vi "1B_AnalyzePulseTrain.vi"(0 "Waveform In":waveform(dbl)={"t0"=timestamp(3433165898.5470004 s since 1904-01-01), "dt"=1e-05, "Y"=array[4250 elements]}, 5 "Repetitions in the Input Waveform":i32, 7 "Pulse Characteristics":T1={"Pulses per Cycle"=2, "Load Resistance (Ohms)"=750.0, "Krec Value"=2, "Recovery Mode (T=Active)"=TRUE, "Target Stim Currents (Amps)"=[]}) -> (2 "Avg. CBC Width":dbl format="%0.2f", 3 "Avg. CBC Amplitude":dbl format="%0.2f", 4 "Stim PW":dbl[](array[numeric]), 6 "Stim Amplitude":dbl[](array[numeric]), 8 "Interphase Delay":dbl[](array[numeric]), 10 "Recovery PW":dbl[](array[numeric]), 12 "Waveform Parameters":T2, 13 "Frequency":dbl, 14 "Recovery Holdoff":dbl[](array[numeric]), 15 "Recovery Amplitude":dbl[](array[numeric]))   [LabVIEW 2010]
uses:
  <vilib>/measure/mamon.llb/Trigger Detection for 1 Channel.vi
  <vilib>/measure/NI_MAPro.lvlib
  <vilib>/Analysis/NI_AALBase.lvlib
panel:
  in  "View":enum32{"View All", "Graph Only"}(tab)
  out "Waveform in ( graph )":waveform(dbl)(graph)
  out "Normalized Waveform":waveform(dbl)(graph)
  out "Offset":dbl
  out "Current in amps":waveform(dbl)(graph)
  # "Remove idle voltage offset\n( if applicable )"
  # "The input waveform should be a capture of the STIM chip output\n(before the cap) when the output is held at 1/2 HVDD by the\nLoad Resistance.  This ensures that passive recovery and CBC\npulses are captured, because they look like pulses pulled to GND."
  # "The elements in these arrays correspond to the pulses per cycle.\nThey are the averages over all the repetitions in the waveform."
  # "Enter Target Current\nfor each in array below"
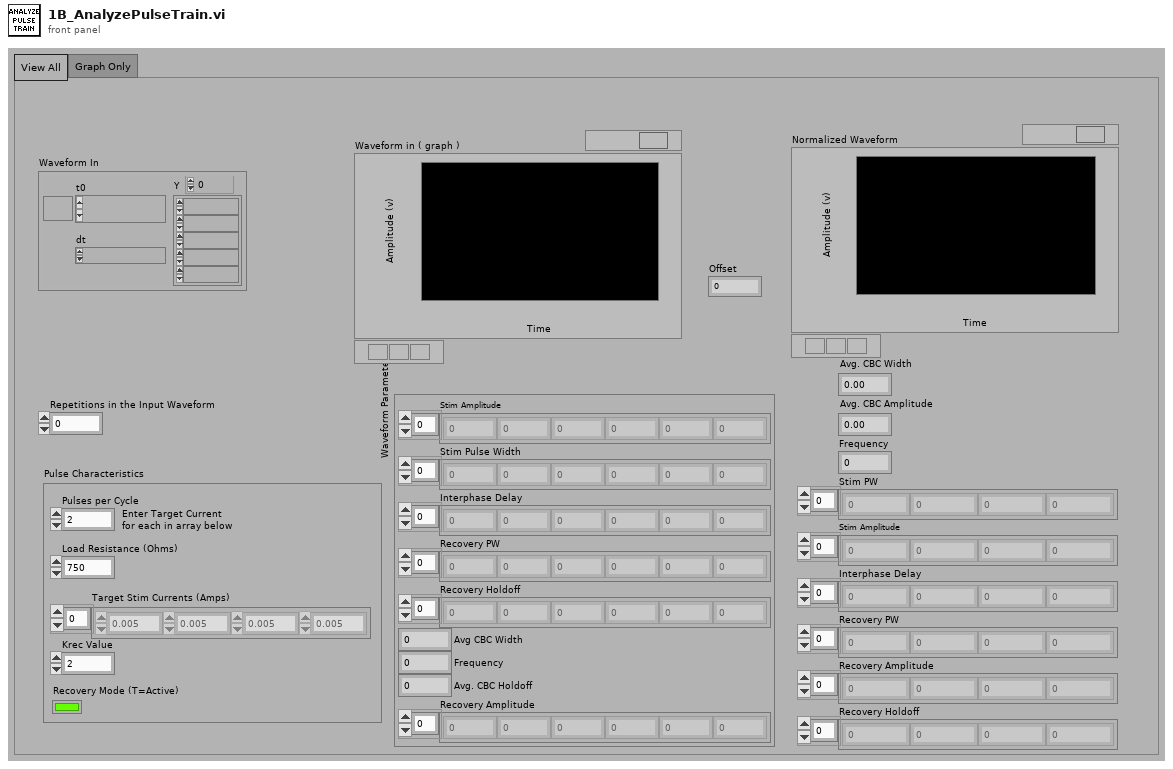
[diagram p1: front panel]
types:
  T1 = cluster{"Pulses per Cycle":i32, "Load Resistance (Ohms)":dbl, "Krec Value":i32, "Recovery Mode (T=Active)":bool, "Target Stim Currents (Amps)":dbl[]}
  T2 = cluster{"Stim Amplitude":dbl[], "Stim Pulse Width":dbl[], "Interphase Delay":dbl[], "Recovery PW":dbl[], "Recovery Holdoff":dbl[], "Avg CBC Width":dbl, "Frequency":dbl, "Avg. CBC Holdoff":dbl, "Recovery Amplitude":dbl[]}
  T3 = cluster{"trigger slope":u16, "Trigger Level":dbl}[]
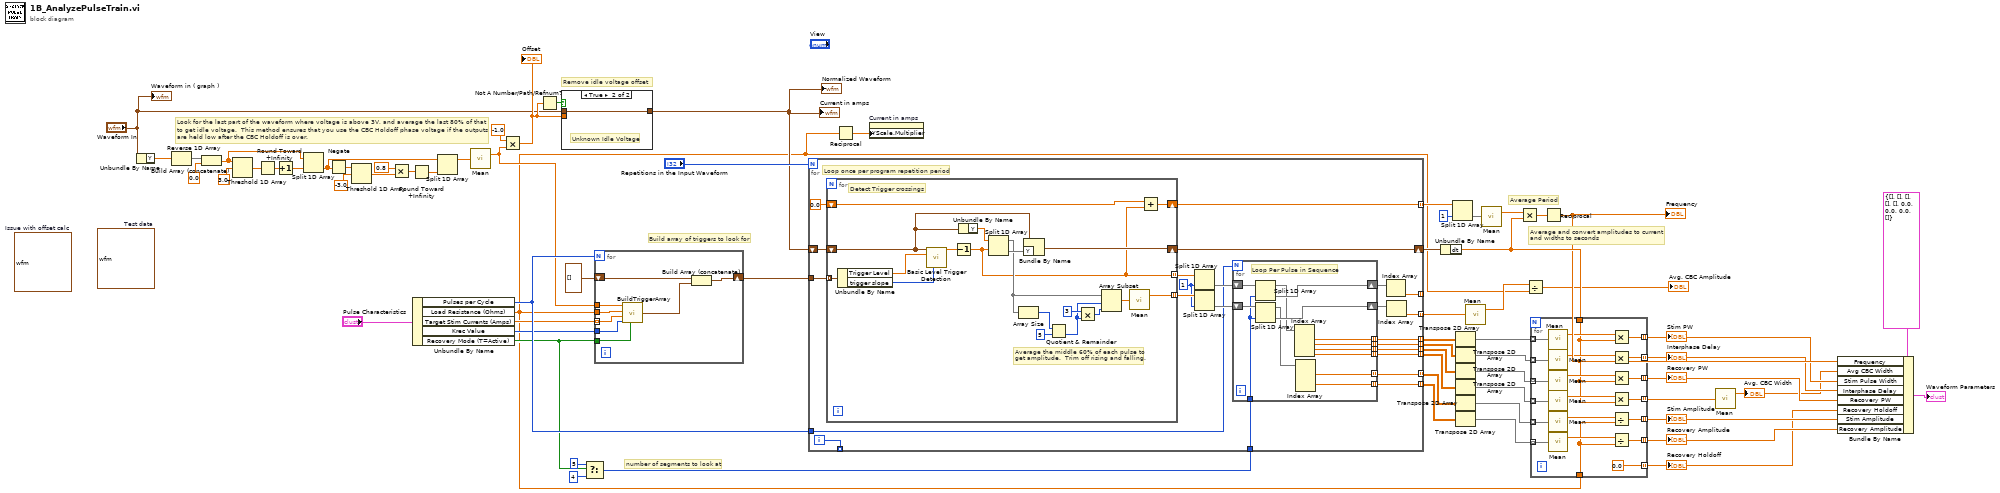
[diagram p0: block diagram]
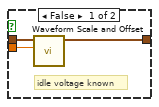
[diagram p2: hidden frame]
diagram:
  (unwired) waveform(dbl) {"t0"=timestamp(3458836317.3280005 s since 1904-01-01), "dt"=1.428e-05, "Y"=array[4000 elements]}  # Issue with offset calc
  (unwired) waveform(dbl) {"t0"=timestamp(3418839276.250478 s since 1904-01-01), "dt"=1e-06, "Y"=[5.0, 5.0, 9.0, 9.0, 9.0, 9.0, 9.0, 9.0, 9.0, 9.0, 5.0, 5.0, 5.0, 3.0, 3.0, 3.0, 3.0, 3.0, 3.0, 3.0, 3.0, 3.0, 3.0, 3.0, 3.0, 3.0, 3.0, 3.0, 3.0, 5.0, 5.0, 5.0, 5.0, 8.0, 8.0, 8.0, 8.0, 8.0, 8.0, 8.0, 8.0, 5.0, 5.0, 5.0, 3.0, 3.0, 3.0, 3.0, 3.0, 3.0, 3.0, 3.0, 3.0, 3.0, 3.0, 3.0, 3.0, 3.0, 3.0, 3.0, 5.0, 5.0, 5.0, 5.0, 0.0, 0.0, 0.0, 0.0, 0.0, 5.0, 5.0, 5.0, 5.0, 5.0, 5.0, 5.0, 5.0, 5.0, 5.0, 5.0, 5.0, 5.0, 5.0, 5.0, 5.0, 5.0, 5.0, 5.0, 5.0, 5.0, 5.0, 5.0, 5.0, 5.0, 5.0, 5.0, 5.0, 5.0, 5.0, 5.0, 5.0, 5.0, 9.0, 9.0, 9.0, 9.0, 9.0, 9.0, 9.0, 9.0, 5.0, 5.0, 5.0, 3.0, 3.0, 3.0, 3.0, 3.0, 3.0, 3.0, 3.0, 3.0, 3.0, 3.0, 3.0, 3.0, 3.0, 3.0, 3.0, 5.0, 5.0, 5.0, 5.0, 8.0, 8.0, 8.0, 8.0, 8.0, 8.0, 8.0, 8.0, 5.0, 5.0, 5.0, 3.0, 3.0, 3.0, 3.0, 3.0, 3.0, 3.0, 3.0, 3.0, 3.0, 3.0, 3.0, 3.0, 3.0, 3.0, 3.0, 5.0, 5.0, 5.0, 5.0, 0.0, 0.0, 0.0, 0.0, 0.0, 5.0, 5.0, 5.0, 5.0, 5.0, 5.0, 5.0, 5.0, 5.0, 5.0, 5.0, 5.0, 5.0, 5.0, 5.0, 5.0, 5.0, 5.0, 5.0, 5.0, 5.0, 5.0, 5.0, 5.0, 5.0, 5.0, 5.0, 5.0, 5.0, 5.0, 5.0, 5.0, 5.0, 9.0, 9.0, 9.0, 9.0, 9.0, 9.0, 9.0, 9.0, 5.0, 5.0, 5.0, 3.0, 3.0, 3.0, 3.0, 3.0, 3.0, 3.0, 3.0, 3.0, 3.0, 3.0, 3.0, 3.0, 3.0, 3.0, 3.0, 5.0, 5.0, 5.0, 5.0, 8.0, 8.0, 8.0, 8.0, 8.0, 8.0, 8.0, 8.0, 5.0, 5.0, 5.0, 3.0, 3.0, 3.0, 3.0, 3.0, 3.0, 3.0, 3.0, 3.0, 3.0, 3.0, 3.0, 3.0, 3.0, 3.0, 3.0, 5.0, 5.0, 5.0, 5.0, 0.0, 0.0, 0.0, 0.0, 0.0, 5.0, 5.0, 5.0, 5.0, 5.0, 5.0, 5.0, 5.0, 5.0, 5.0, 5.0, 5.0, 5.0, 5.0, 5.0, 5.0, 5.0, 5.0, 5.0, 5.0, 5.0, 5.0, 5.0, 5.0, 5.0, 5.0, 5.0, 5.0, 5.0, 5.0, 5.0, 5.0, 5.0, 9.0, 9.0, 9.0, 9.0, 9.0, 9.0, 9.0, 9.0, 5.0, 5.0, 5.0, 3.0, 3.0, 3.0, 3.0, 3.0, 3.0, 3.0, 3.0, 3.0, 3.0, 3.0, 3.0, 3.0, 3.0, 3.0, 3.0, 5.0, 5.0, 5.0, 5.0, 8.0, 8.0, 8.0, 8.0, 8.0, 8.0, 8.0, 8.0, 5.0, 5.0, 5.0, 3.0, 3.0, 3.0, 3.0, 3.0, 3.0, 3.0, 3.0, 3.0, 3.0, 3.0, 3.0, 3.0, 3.0, 3.0, 3.0, 5.0, 5.0, 5.0, 5.0, 0.0, 0.0, 0.0, 0.0, 0.0, 5.0, 5.0, 5.0, 5.0, 5.0, 5.0, 5.0, 5.0, 5.0, 5.0, 5.0, 5.0, 5.0, 5.0, 5.0, 5.0, 5.0, 5.0, 5.0, 5.0, 5.0, 5.0, 5.0, 5.0, 5.0, 5.0, 5.0, 5.0, 5.0, 5.0, 5.0, 5.0, 5.0, 9.0, 9.0, 9.0, 9.0, 9.0, 9.0, 9.0, 9.0, 5.0, 5.0, 5.0, 3.0, 3.0, 3.0, 3.0, 3.0, 3.0, 3.0, 3.0, 3.0, 3.0, 3.0, 3.0, 3.0, 3.0, 3.0, 3.0, 5.0, 5.0, 5.0, 5.0, 8.0, 8.0, 8.0, 8.0, 8.0, 8.0, 8.0, 8.0, 5.0, 5.0, 5.0, 3.0, 3.0, 3.0, 3.0, 3.0, 3.0, 3.0, 3.0, 3.0, 3.0, 3.0, 3.0, 3.0, 3.0, 3.0, 3.0, 5.0, 5.0, 5.0, 5.0, 0.0, 0.0, 0.0, 0.0, 0.0, 5.0, 5.0, 5.0, 5.0, 5.0, 5.0, 5.0, 5.0, 5.0, 5.0, 5.0, 5.0, 5.0, 5.0, 5.0, 5.0, 5.0, 5.0, 5.0, 5.0, 5.0, 5.0, 5.0, 5.0, 5.0, 5.0, 5.0, 5.0, 5.0, 5.0, 5.0, 5.0, 5.0, 5.0]}  # Test data
  # "number of segments to look at"
  # "Look for the last part of the waveform where voltage is above 3V, and average the last 80% of that\nto get idle voltage.  This method ensures that you use the CBC Holdoff phase voltage if the outputs\nare held low after the CBC Holdoff is over."
  # "Average Period"
  # "Average and convert amplitudes to current\nand widths to seconds"
  # "Build array of triggers to look for"
  # "Remove idle voltage offset"
  n1 = Unbundle By Name("Waveform In") -> ("Y"=w2:dbl[])
  n2 = Reverse 1D Array(array=w2) -> (reversed array=w31:dbl[])
  n3 = Build Array (concatenate)(w31, 0.0 ("y")) -> (w5:dbl[])
  n4 = Threshold 1D Array(2:3.0 ("y"), 3:w5) -> (0:w28:dbl)  [unwired: 1 in]
  n5 = Round Toward +Infinity(x=w28) -> (ceil(x): smallest int >= x=w27:dbl)
  n6 = Increment(x=w27) -> (x+1=w20:dbl)
  n7 = Split 1D Array(array=w5, index=w20) -> (second subarray=w4:dbl[])  [unwired: 1 out]
  n8 = Negate(x=w4) -> (-x=w25:dbl[])
  n9 = Threshold 1D Array(2:-3.0 ("y"), 3:w25) -> (0:w24:dbl)  [unwired: 1 in]
  n10 = Multiply(x=0.8, y=w24) -> (x*y=w22:dbl)
  n11 = Round Toward +Infinity(x=w22) -> (ceil(x): smallest int >= x=w21:dbl)
  n12 = Unbundle By Name("Pulse Characteristics") -> ("Pulses per Cycle"=w52:i32, "Load Resistance (Ohms)"=w9:dbl, "Target Stim Currents (Amps)"=w51:dbl[], "Krec Value"=w50:i32, "Recovery Mode (T=Active)"=w14:bool)
  n13 = Split 1D Array(array=w4, index=w21) -> (first subarray=w3:dbl[])  [unwired: 1 out]
  n14 = call <vilib>:"Mean.vi"("X"=w3) -> ("mean"=w15:dbl)  [unwired: 1 out]
  n15 = Multiply(x=-1.0, y=w15) -> (x*y=w7:dbl)
  "Offset" <- w7
  n16 = Not A Number/Path/Refnum?(number/path/refnum=w7) -> (NaN/Path/Refnum?=w6:bool)
  n17 = case shown="True" w6 {
    tunnel: [w71 w72] -> w10
    tunnel: "Waveform In" -> [w70 w72]
    tunnel: w7 -> [w69 _]
    frame False {
      # "idle voltage known"
      n18 = call <vilib>:"Waveform Scale and Offset.vi"("offset"=w69, "waveform in"=w70) -> ("waveform out"=w71:waveform(dbl))  [unwired: 8 in, 1 out]
    }
    frame True {
      # "Unknown Idle Voltage"
    }
  }
  "Normalized Waveform" <- w10
  "Current in amps" <- w10
  n19 = Select(t=5, s=w14, f=4 ("index")) -> (s? t:f=w12:i32)
  n20 = for {
    N: w52 -> [_]
    shift-right: [w80] -> w19
    shift-left: T3 [] -> [w79]
    tunnel: w15 -> [w78]
    tunnel: w14 -> [w77]
    tunnel: w9 -> [w76]
    tunnel: w51 -> [w75] mode=indexing
    tunnel: w50 -> [w74]
    n21 = call "BuildTriggerArray.vi"("CBC Trigger Level"=w78, "Load Resistance (Ohms)"=w76, "Target Stim Current (Amps)"=w75, "Krec Value"=w74, "Recovery Mode (T=Active)"=w77) -> ("Pulse Triggers"=w73:T3)
    n22 = Build Array (concatenate)(w79, w73) -> (w80:T3)
  }
  n23 = for {
    N: "Repetitions in the Input Waveform" -> [_]
    tunnel: w19 -> [w103]
    shift-right: [w99] -> w48
    shift-left: w10 -> [w102]
    tunnel: w52 -> [w96]
    tunnel: [w93] -> _ mode=indexing
    tunnel: [w92] -> w65 mode=indexing
    tunnel: [w91] -> w64 mode=indexing
    tunnel: [w90] -> w63 mode=indexing
    tunnel: [w89] -> w62 mode=indexing
    tunnel: [w88] -> w61 mode=indexing
    tunnel: [w87] -> w60 mode=indexing
    tunnel: [w86] -> w59 mode=indexing
    tunnel: [w83] -> w46 mode=indexing
    tunnel: w12 -> [w82]
    tunnel: [w81] -> _ mode=indexing
    i -> [w81]
    w100 = 1 ("index")
    # "Loop once per program repetition period"
    n24 = for {
      tunnel: w103 -> [w135] mode=indexing
      shift-right: [w121] -> w99
      shift-left: w102 -> [w130]
      tunnel: [w122] -> w101 mode=indexing
      tunnel: [w117] -> w84 mode=indexing
      shift-right: [w120] -> w83
      shift-left: 0.0 -> [w119]
      # "Detect Trigger crossings"
      # "Average the middle 60% of each pulse to\nget amplitude.  Trim off rising and falling."
      n25 = Unbundle By Name(w135) -> ("Trigger Level"=w134:dbl, "trigger slope"=w133:u16)
      n26 = call-poly <vilib>:"Basic Level Trigger Detection.vi"("signal in"=w130, "level"=w134, "trigger slope"=w133) -> ("trigger location"=w118:dbl)  [unwired: 10 in, 2 out]
      n27 = Decrement(x=w118) -> (x-1=w117:dbl)
      n28 = Unbundle By Name(w130) -> ("Y"=w132:dbl[])
      n29 = Split 1D Array(array=w132, index=w117) -> (first subarray=w124:dbl[], second subarray=w131:dbl[])
      n30 = Array Size(array=w124) -> (size(s)=w129:i32)
      n31 = Bundle By Name(cluster=w130, "Y"=w131) -> (w121:waveform(dbl))
      n32 = Quotient & Remainder(x=w129, y=5) -> (floor(x/y)=w126:i32)  [unwired: 1 out]
      n33 = Multiply(x=3, y=w126) -> (x*y=w125:i32)
      n34 = Array Subset(array=w124, index=w126, length=w125) -> (w123:dbl[])
      n35 = call <vilib>:"Mean.vi"("X"=w123) -> ("mean"=w122:dbl)  [unwired: 1 out]
      n36 = Add(x=w119, y=w117) -> (x+y=w120:dbl)
    }
    n37 = Split 1D Array(array=w84, index=w100) -> (second subarray=w98:dbl[])  [unwired: 1 out]
    n38 = Split 1D Array(array=w101, index=w100) -> (second subarray=w97:dbl[])  [unwired: 1 out]
    n39 = for {
      N: w96 -> [_]
      shift-right: [w114] -> w95
      shift-left: w98 -> [w116]
      shift-right: [w113] -> w94
      shift-left: w97 -> [w115]
      tunnel: [w110] -> w91 mode=indexing
      tunnel: [w109] -> w90 mode=indexing
      tunnel: [w108] -> w89 mode=indexing
      tunnel: [w107] -> w88 mode=indexing
      tunnel: [w106] -> w87 mode=indexing
      tunnel: [w105] -> w86 mode=indexing
      tunnel: w82 -> [w104]
      # "Loop Per Pulse in Sequence"
      n40 = Split 1D Array(array=w116, index=w104) -> (first subarray=w112:dbl[], second subarray=w114:dbl[])
      n41 = Split 1D Array(array=w115, index=w104) -> (first subarray=w111:dbl[], second subarray=w113:dbl[])
      n42 = Index Array(array=w112) -> (element #1=w110:dbl, element #2=w109:dbl, element #3=w108:dbl, element #4=w107:dbl)  [unwired: 4 in]
      n43 = Index Array(array=w111) -> (element #1=w106:dbl, element #3=w105:dbl)  [unwired: 4 in, 2 out]
    }
    n44 = Index Array(array=w95) -> (element=w93:dbl)  [unwired: 1 in]
    n45 = Index Array(array=w94) -> (element=w92:dbl)  [unwired: 1 in]
  }
  n46 = Reciprocal(x=w9) -> (1/x=w8:dbl)
  n47 = property on="Current in amps" class="WFGraph (strict)"("YScale.Multiplier"=w8) -> ()  [unwired: 2 in, 2 out]
  n48 = Unbundle By Name(w48) -> ("dt"=w43:dbl)
  n49 = Split 1D Array(array=w46, index=1) -> (second subarray=w45:dbl[])  [unwired: 1 out]
  n50 = Transpose 2D Array(2D array=w64) -> (transposed array=w58:dbl[][])
  n51 = Transpose 2D Array(2D array=w63) -> (transposed array=w57:dbl[][])
  n52 = Transpose 2D Array(2D array=w62) -> (transposed array=w56:dbl[][])
  n53 = Transpose 2D Array(2D array=w61) -> (transposed array=w55:dbl[][])
  n54 = Transpose 2D Array(2D array=w60) -> (transposed array=w54:dbl[][])
  n55 = Transpose 2D Array(2D array=w59) -> (transposed array=w53:dbl[][])
  n56 = call <vilib>:"Mean.vi"("X"=w65) -> ("mean"=w47:dbl)  [unwired: 1 out]
  n57 = call <vilib>:"Mean.vi"("X"=w45) -> ("mean"=w44:dbl)  [unwired: 1 out]
  n58 = Multiply(x=w44, y=w43) -> (x*y=w42:dbl)
  n59 = Divide(x=w47, y=w9) -> (x/y=→"Avg. CBC Amplitude":dbl)
  n60 = for {
    tunnel: w58 -> [w156] mode=indexing
    tunnel: w57 -> [w155] mode=indexing
    tunnel: w56 -> [w154] mode=indexing
    tunnel: w55 -> [w153] mode=indexing
    tunnel: w54 -> [w152] mode=indexing
    tunnel: w53 -> [w151] mode=indexing
    tunnel: [w150] -> w37 mode=indexing
    tunnel: [w149] -> w36 mode=indexing
    tunnel: [w148] -> w35 mode=indexing
    tunnel: [w147] -> w17 mode=indexing
    tunnel: [w146] -> w34 mode=indexing
    tunnel: [w145] -> w33 mode=indexing
    tunnel: w43 -> [w138]
    tunnel: w9 -> [w137]
    tunnel: [0.0 ("Load Resistance (Ohms)")] -> w18 mode=indexing
    n61 = call <vilib>:"Mean.vi"("X"=w156) -> ("mean"=w143:dbl)  [unwired: 1 out]
    n62 = call <vilib>:"Mean.vi"("X"=w155) -> ("mean"=w142:dbl)  [unwired: 1 out]
    n63 = call <vilib>:"Mean.vi"("X"=w154) -> ("mean"=w141:dbl)  [unwired: 1 out]
    n64 = call <vilib>:"Mean.vi"("X"=w153) -> ("mean"=w140:dbl)  [unwired: 1 out]
    n65 = call <vilib>:"Mean.vi"("X"=w152) -> ("mean"=w139:dbl)  [unwired: 1 out]
    n66 = call <vilib>:"Mean.vi"("X"=w151) -> ("mean"=w144:dbl)  [unwired: 1 out]
    n67 = Multiply(x=w143, y=w138) -> (x*y=w150:dbl)
    n68 = Multiply(x=w142, y=w138) -> (x*y=w149:dbl)
    n69 = Multiply(x=w141, y=w138) -> (x*y=w148:dbl)
    n70 = Multiply(x=w140, y=w138) -> (x*y=w147:dbl)
    n71 = Divide(x=w139, y=w137) -> (x/y=w146:dbl)
    n72 = Divide(x=w144, y=w137) -> (x/y=w145:dbl)
  }
  "Stim PW" <- w37
  "Interphase Delay" <- w36
  "Recovery PW" <- w35
  "Recovery Holdoff" <- w18
  "Stim Amplitude" <- w34
  "Recovery Amplitude" <- w33
  n73 = Reciprocal(x=w42) -> (1/x=w39:dbl)
  "Frequency" <- w39
  n74 = call <vilib>:"Mean.vi"("X"=w17) -> ("mean"=w16:dbl)  [unwired: 1 out]
  "Avg. CBC Width" <- w16
  n75 = Bundle By Name(cluster=T2 {"Stim Amplitude"=[], "Stim Pulse Width"=[], "Interphase Delay"=[], "Recovery PW"=[], "Recovery Holdoff"=[], "Avg CBC Width"=0.0, "Frequency"=0.0, "Avg. CBC Holdoff"=0.0, "Recovery Amplitude"=[]} ("Pulse Train Parameters"), "Frequency"=w39, "Avg CBC Width"=w16, "Stim Pulse Width"=w37, "Interphase Delay"=w36, "Recovery PW"=w35, "Recovery Holdoff"=w18, "Stim Amplitude"=w34, "Recovery Amplitude"=w33) -> (→"Waveform Parameters":T2)
  "Waveform in ( graph )" <- "Waveform In"
